vi "ServotoPWM.vi"(8 "freq [Hz]":dbl, 10 "Duty In":dbl) -> (0 "Duty Cycle":dbl, 1 "Duty Cycle %":dbl, 2 "Pulse Width":dbl)   [LabVIEW 2013]
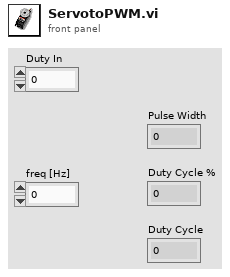
[diagram p1: front panel]
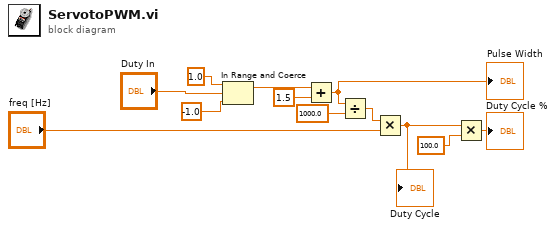
[diagram p0: block diagram]
diagram:
  n1 = In Range and Coerce(upper limit=1.0, x="Duty In", lower limit=-1.0 ("x")) -> (coerced(x)=w2:dbl)  [unwired: 1 out]
  n2 = Add(x=w2, y=1.5) -> (x+y=w6:dbl)
  "Pulse Width" <- w6
  n3 = Divide(x=w6, y=1000.0) -> (x/y=w9:dbl)
  n4 = Multiply(x=w9, y="freq [Hz]") -> (x*y=w12:dbl)
  "Duty Cycle" <- w12
  n5 = Multiply(x=w12, y=100.0) -> (x*y=→"Duty Cycle %":dbl)
